vi "TreeItem.Property.Get.vi"(6 "Custom Device Path":string, 8 "error in (no error)":errorcluster, 9 "Default Value":variant, 10 "Property Name":string, 11 "Basenode":refnum<k24>) -> (0 "error out":errorcluster, 1 "Variant":variant, 2 "Found?":bool, 3 "Basenode":refnum<k24>)   [LabVIEW 2017, in "Advanced System Definition.lvlib"]
uses:
  SysDef API/Advanced System Definition.lvlib
  NationalInstruments.VeriStand.SystemStorage
  _Types/Property.DependentFile.ctl
  NationalInstruments.VeriStand
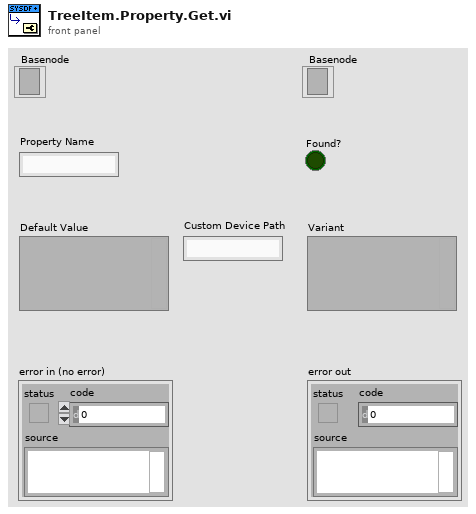
[diagram p1: front panel]
types:
  T1 = typedef "Advanced System Definition.lvlib/Property.DependentFile.ctl" = cluster{"Original Path":path, "Version":string, "RTDestination":path, "ForceDownload":bool, "SupportedTarget":string, "MD5":string}
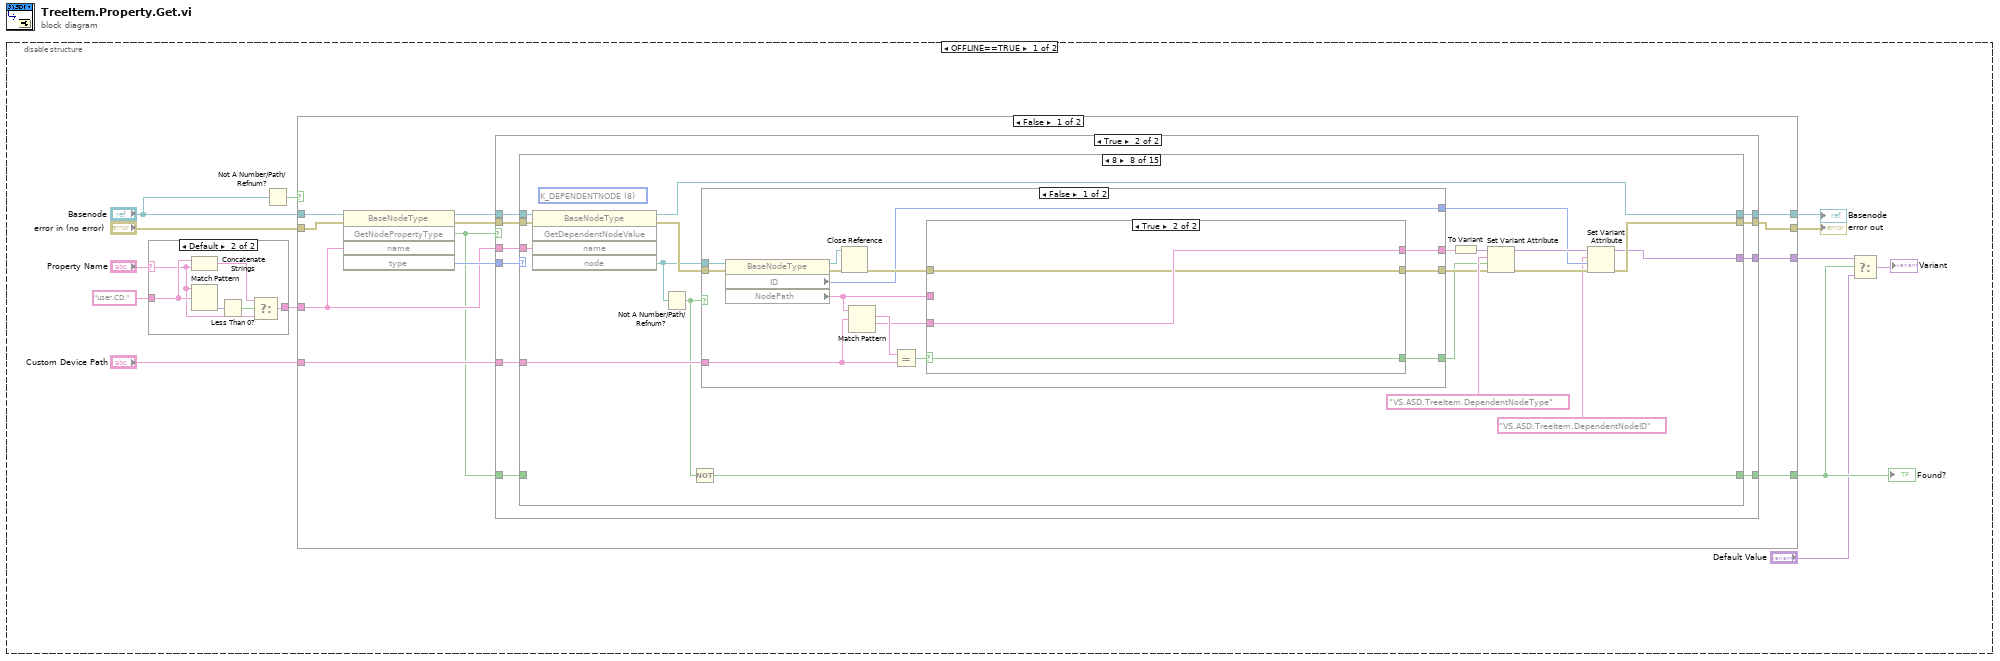
[diagram p0: block diagram]
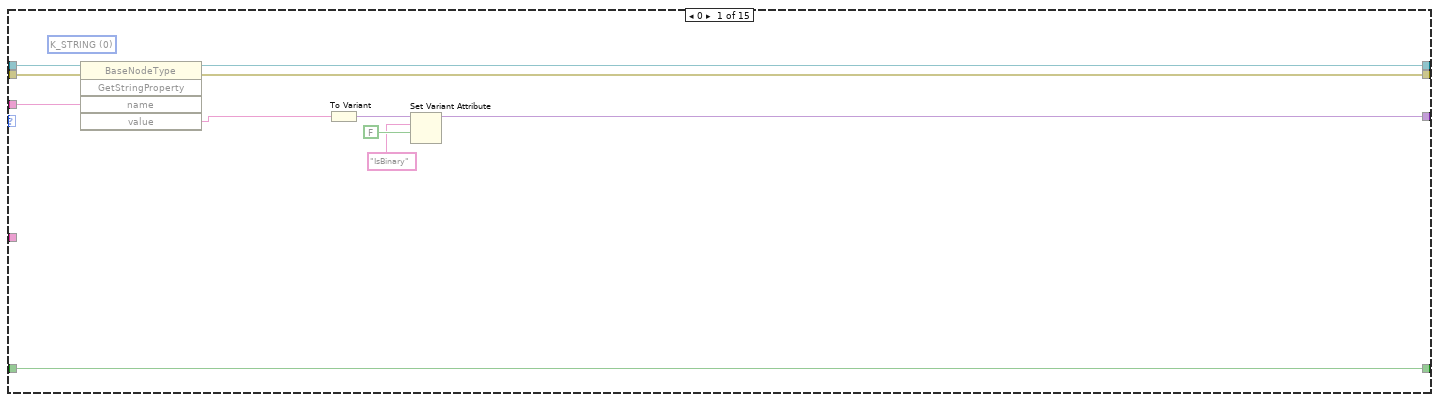
[diagram p4: hidden frame]
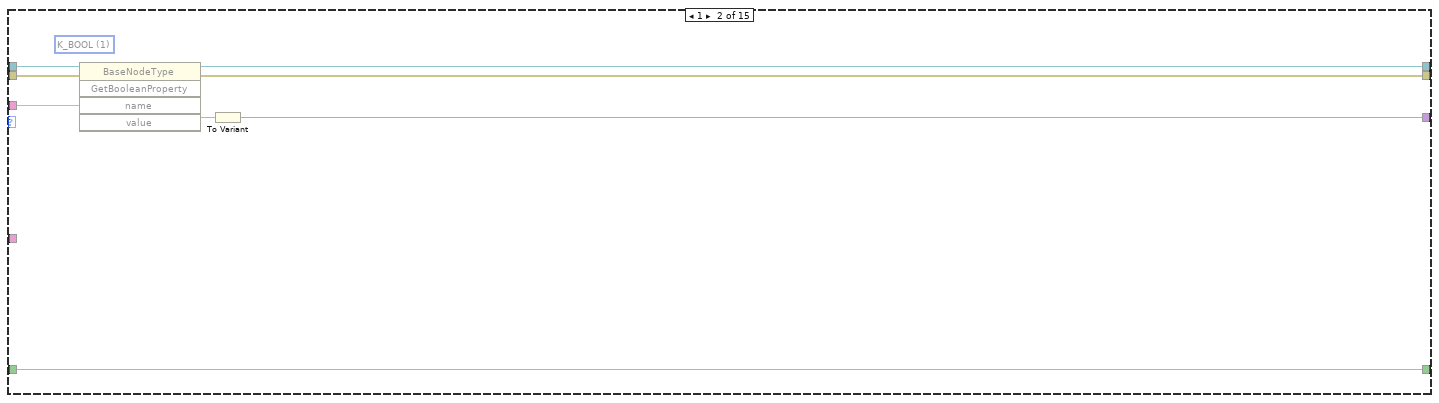
[diagram p5: hidden frame]
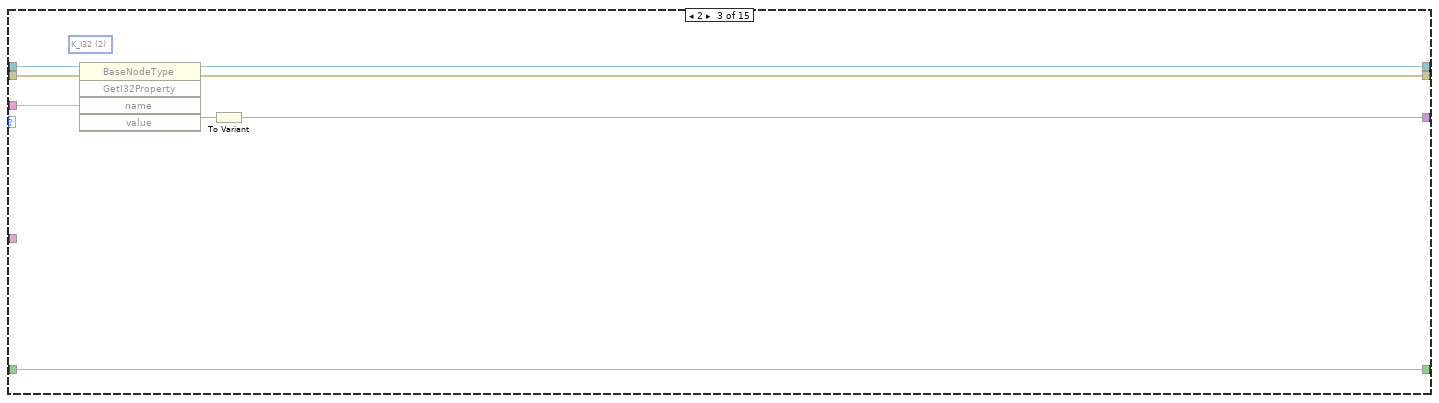
[diagram p6: hidden frame]
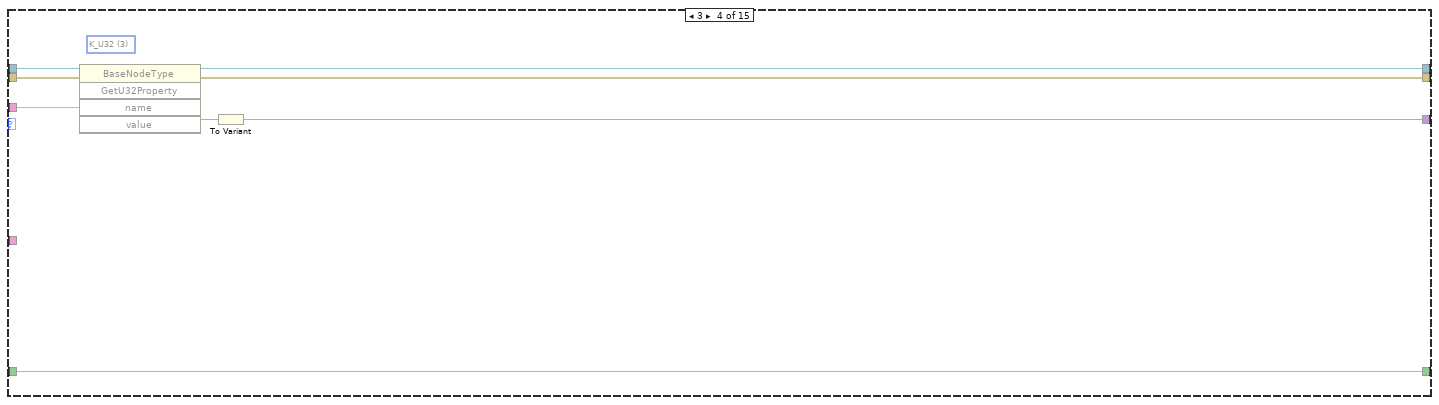
[diagram p7: hidden frame]
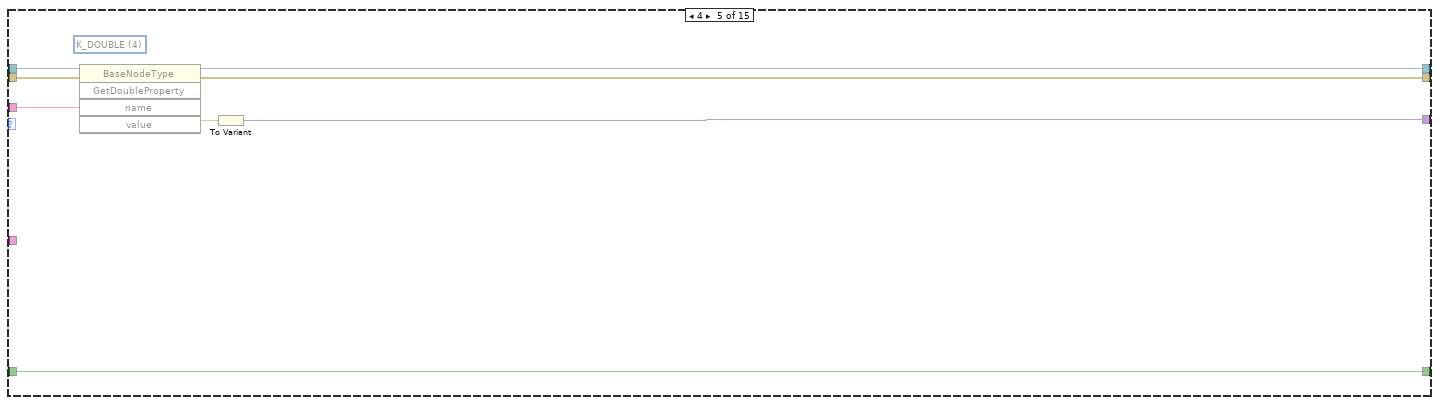
[diagram p8: hidden frame]
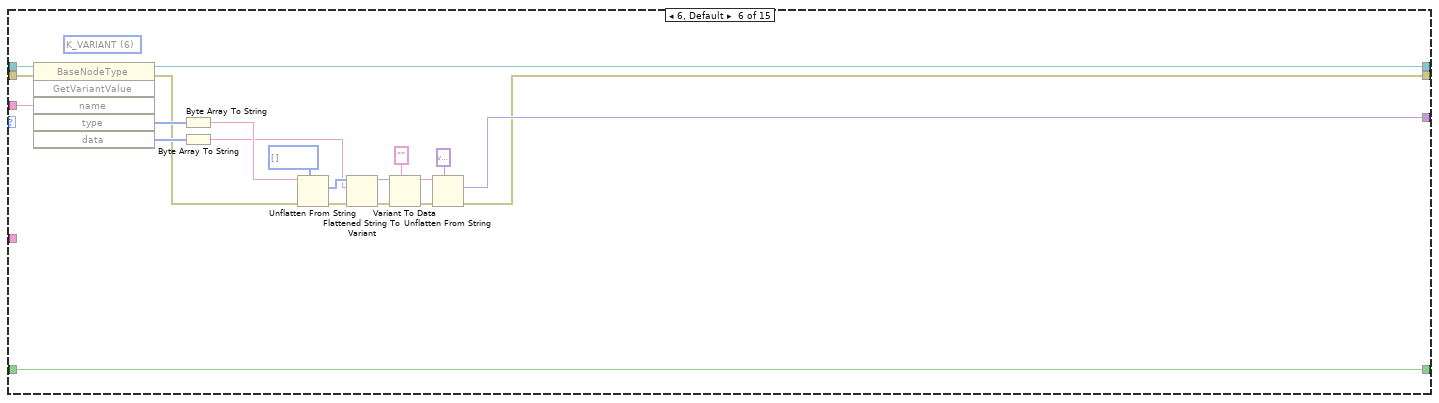
[diagram p9: hidden frame]
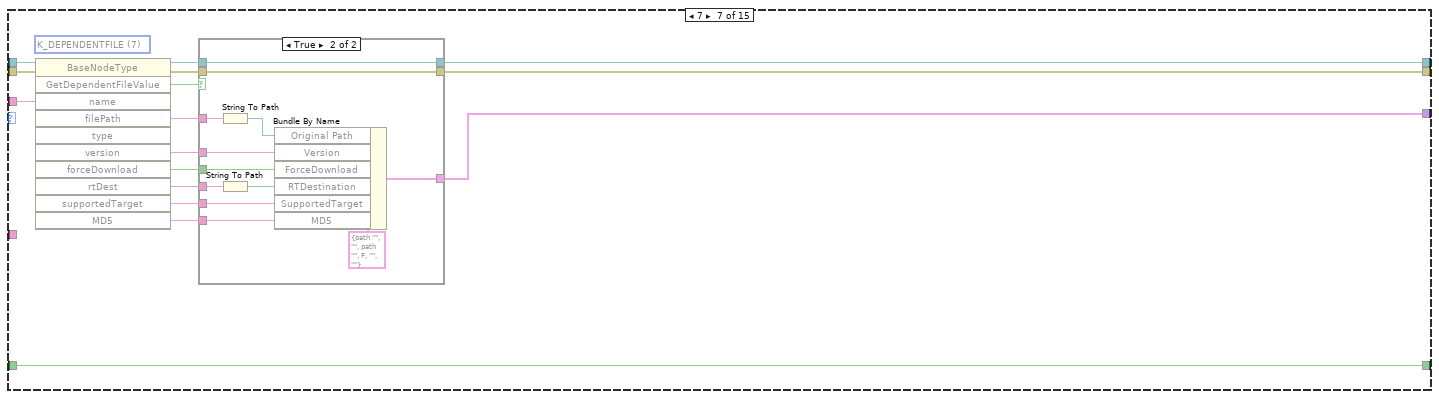
[diagram p10: hidden frame]
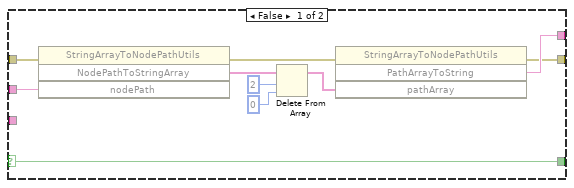
[diagram p12: hidden frame]
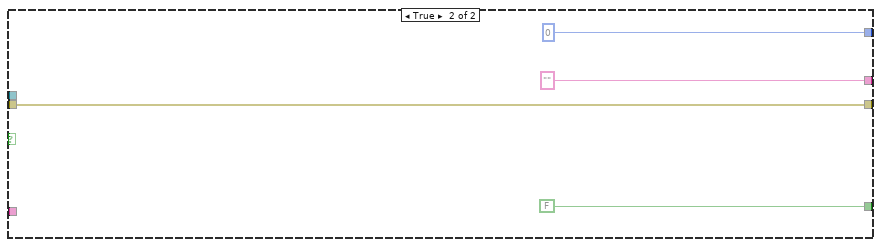
[diagram p13: hidden frame]
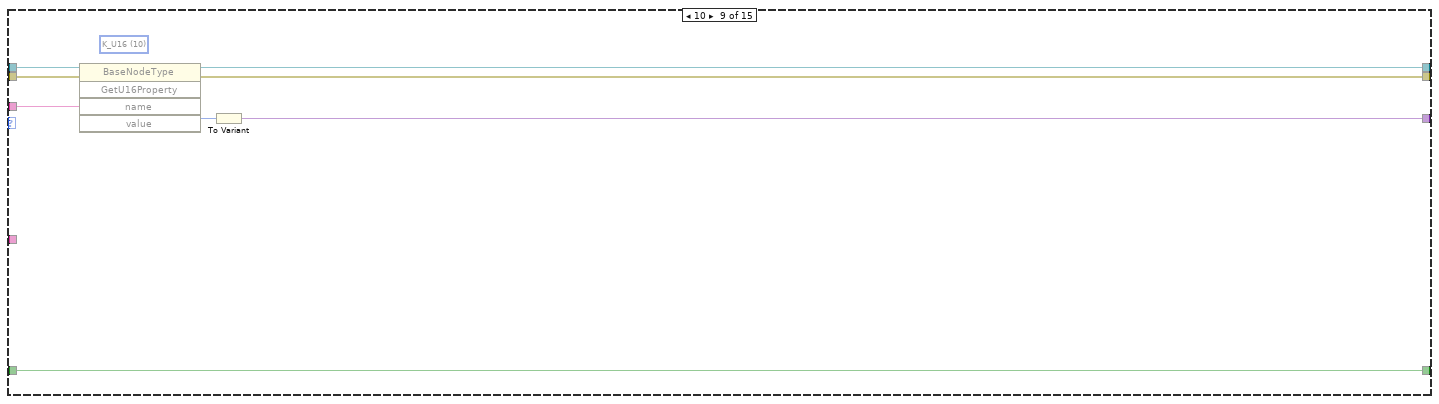
[diagram p14: hidden frame]
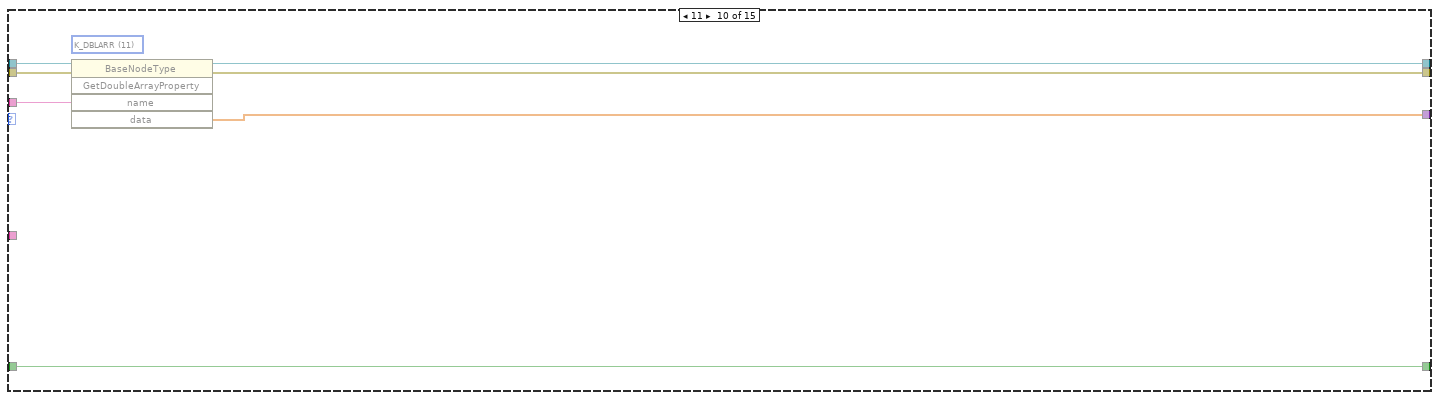
[diagram p15: hidden frame]
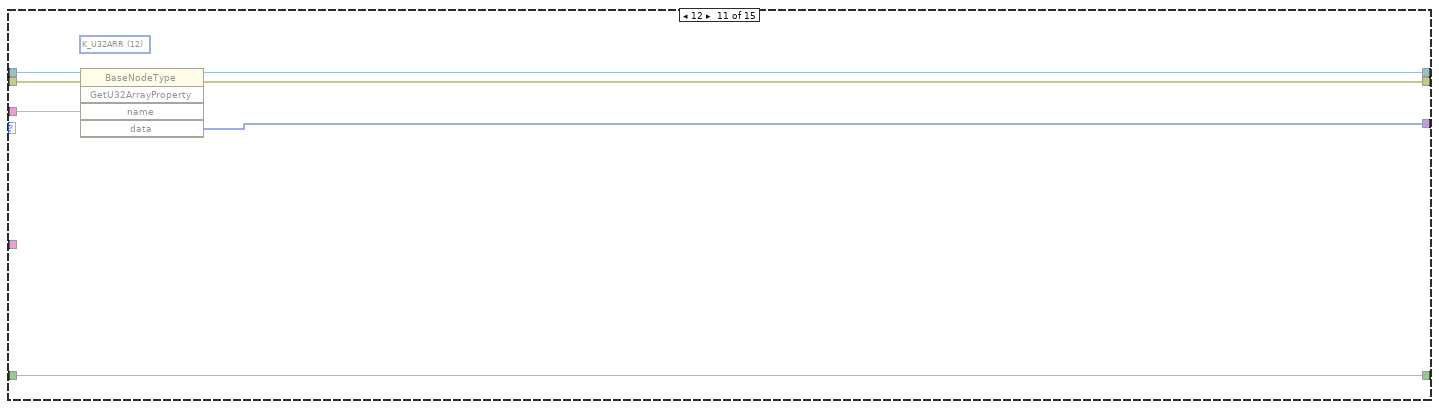
[diagram p16: hidden frame]
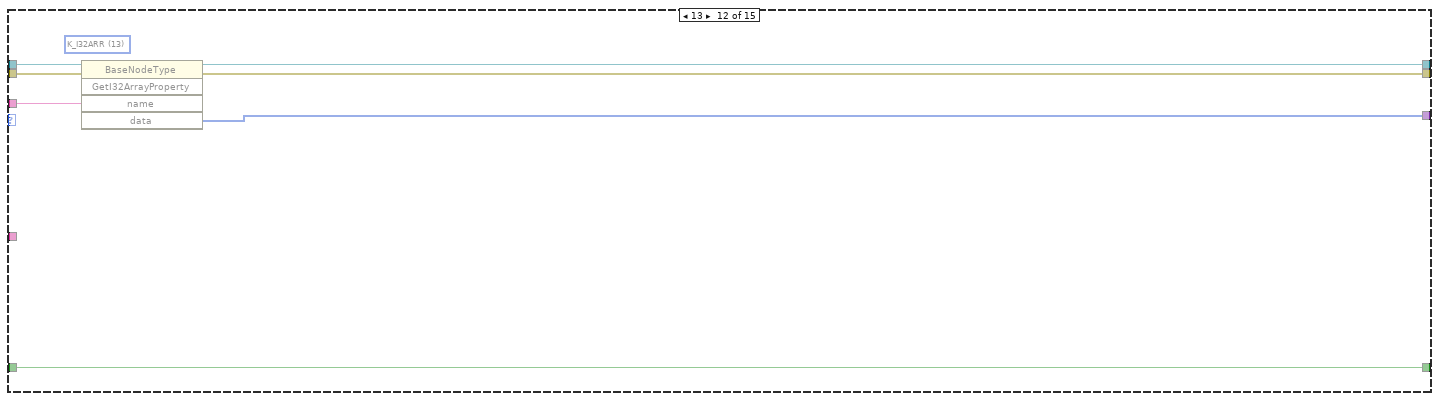
[diagram p17: hidden frame]
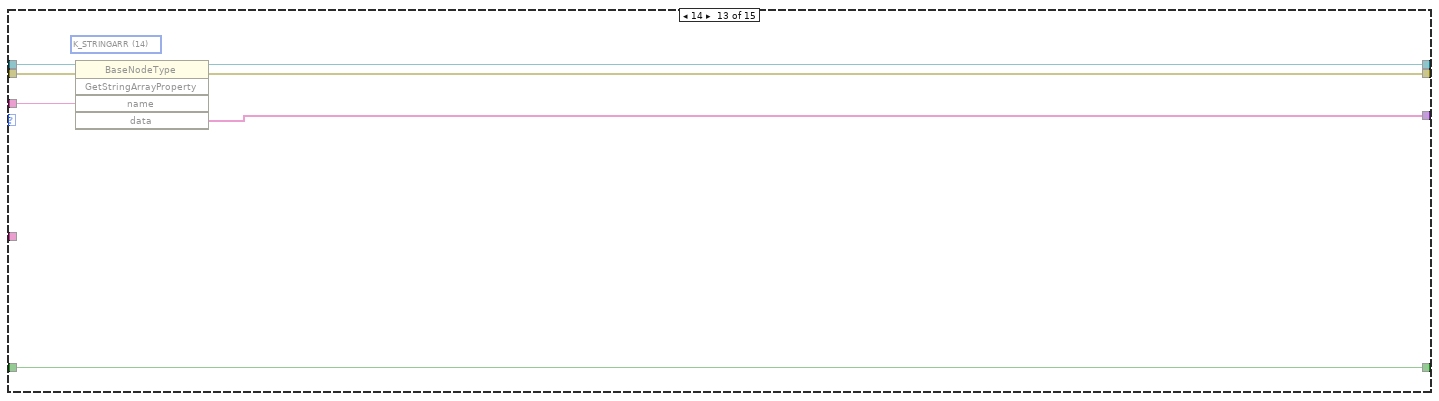
[diagram p18: hidden frame]
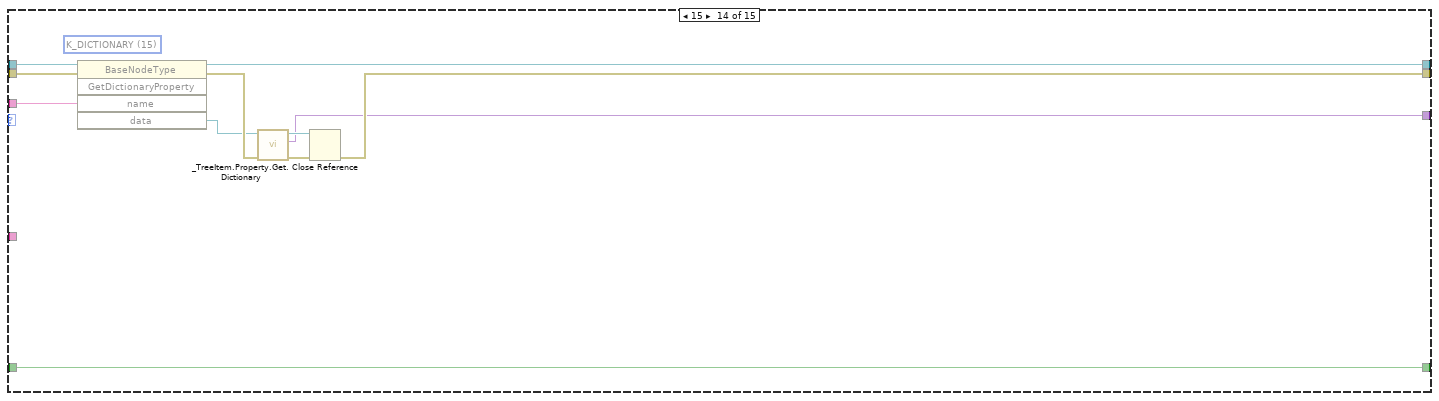
[diagram p19: hidden frame]
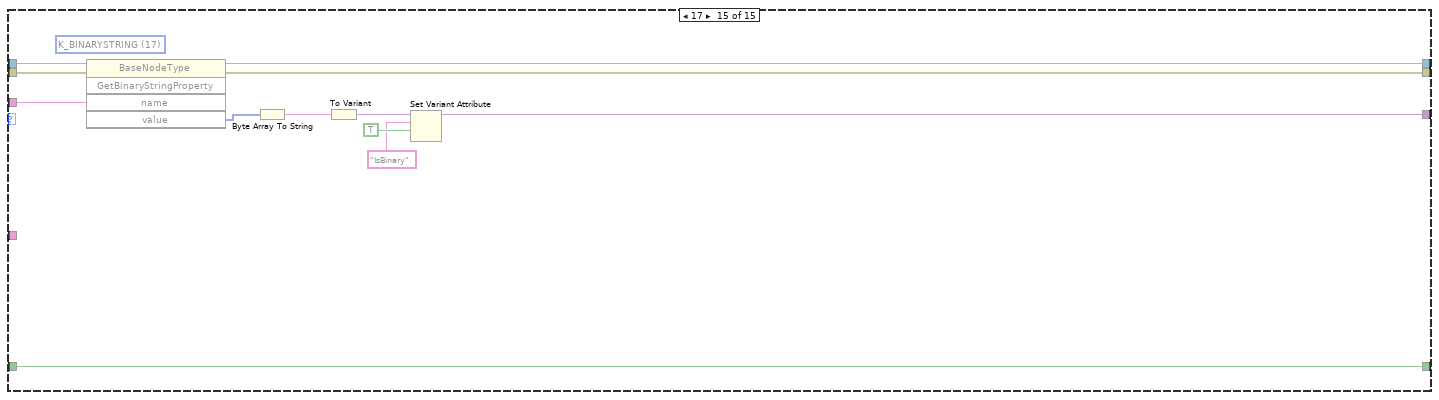
[diagram p20: hidden frame]
diagram:
  n1 = disable-structure shown="OFFLINE==TRUE" {
    frame condition #0 {
      n2 = case shown="Default" "Property Name" {
        selector: "Property Name" -> [w14 w15]
        tunnel: "user.CD." ("regular expression") -> [_ w18]
        tunnel: [w14 w16] -> w3
        frame "Value Table" {
        }
        frame Default {
          n3 = Concatenate Strings(w18, w15) -> (w19:string)
          n4 = Match Pattern(string=w15, regular expression=w18) -> (offset past match=w20:i32)  [unwired: 1 in, 3 out]
          n5 = Less Than 0?(x=w20) -> (x < 0?=w17:bool)
          n6 = Select(t=w19, s=w17, f=w15) -> (s? t:f=w16:string)
        }
      }
      n7 = Not A Number/Path/Refnum?(number/path/refnum="Basenode") -> (NaN/Path/Refnum?=w13:bool)
      n8 = case shown="False" w13 {
        tunnel: w3 -> [w24 _]
        tunnel: "Basenode" -> [w32 w251]
        tunnel: "error in (no error)" -> [w31 w250]
        tunnel: [w21 _] -> w10
        tunnel: [w27 _] -> w9
        tunnel: [w26 w251] -> w6
        tunnel: [w25 w250] -> w5
        tunnel: "Custom Device Path" -> [w23 _]
        frame False {
          n9 = invoke class="BaseNodeType" method="GetNodePropertyType"(reference=w32, error in=w31, "name"=w24) -> (reference out=w28:refnum<k24>, error out=w30:errorcluster, "GetNodePropertyType"=w22:bool, "type"=w29:i32)  [unwired: 2 in, 1 out]
          n10 = case shown="True" w22 {
            tunnel: [w34 w45] -> w26
            tunnel: [w35 w44] -> w25
            tunnel: [_ w43] -> w27
            tunnel: w30 -> [w35 w42]
            tunnel: w29 -> [_ w41]
            tunnel: w28 -> [w34 w40]
            tunnel: w24 -> [_ w39]
            tunnel: w23 -> [_ w38]
            tunnel: [w33 w37] -> w21
            tunnel: w22 -> [w33 w36]
            frame False {
            }
            frame True {
              n11 = case shown="8" w41 {
                tunnel: [w56 w64 w72 w80 w88 w109 w112 w156 w198 w205 w212 w219 w222 w236 w244] -> w45
                tunnel: w42 -> [w55 w63 w71 w79 w87 w108 w121 w159 w197 w204 w211 w218 w226 w237 w248]
                tunnel: [w54 w62 w70 w78 w86 w91 w113 w144 w196 w203 w210 w217 w225 w231 w245] -> w44
                tunnel: [w47 w60 w68 w76 w84 w92 w111 w142 w194 w202 w209 w216 w224 w229 w239] -> w43
                tunnel: w40 -> [w52 w59 w66 w74 w82 w107 w122 w158 w193 w200 w208 w215 w221 w235 w249]
                tunnel: w39 -> [w53 w58 w67 w75 w83 w106 w120 w157 w192 w201 w207 w214 w223 w228 w247]
                tunnel: w38 -> [_ _ _ _ _ _ _ w151 _ _ _ _ _ _ _]
                tunnel: [w46 w57 w65 w73 w81 w89 w110 w146 w191 w199 w206 w213 w220 w227 w238] -> w37
                tunnel: w36 -> [w46 w57 w65 w73 w81 w89 w110 _ w191 w199 w206 w213 w220 w227 w238]
                frame 0 {
                  (unwired) 0 items=["K_STRING", "K_BOOL", "K_I32", "K_U32", "K_DOUBLE", "K_U64", "K_VARIANT", "K_DEPENDENTFILE", "K_DEPENDENTNODE", "K_DATASOURCENODE", "K_U16", "K_DBLARR", "K_U32ARR", "K_I32ARR", "K_STRINGARR", "K_DICTIONARY", "K_DICTIONARYARR"] ("type")
                  n12 = invoke class="BaseNodeType" method="GetStringProperty"(reference=w52, error in=w55, "name"=w53) -> (reference out=w56:refnum<k24>, error out=w54:errorcluster, "value"=w48:string)  [unwired: 2 in, 2 out]
                  n13 = To Variant(anything=w48) -> (Variant=w49:variant)
                  n14 = Set Variant Attribute(Variant=w49, name="IsBinary", value=FALSE ("Set String as Binary")) -> (Variant out=w47:variant)  [unwired: 1 in, 2 out]
                }
                frame 1 {
                  (unwired) 1 items=["K_STRING", "K_BOOL", "K_I32", "K_U32", "K_DOUBLE", "K_U64", "K_VARIANT", "K_DEPENDENTFILE", "K_DEPENDENTNODE", "K_DATASOURCENODE", "K_U16", "K_DBLARR", "K_U32ARR", "K_I32ARR", "K_STRINGARR", "K_DICTIONARY", "K_DICTIONARYARR"] ("type")
                  n15 = invoke class="BaseNodeType" method="GetBooleanProperty"(reference=w59, error in=w63, "name"=w58) -> (reference out=w64:refnum<k24>, error out=w62:errorcluster, "value"=w61:bool)  [unwired: 2 in, 2 out]
                  n16 = To Variant(anything=w61) -> (Variant=w60:variant)
                }
                frame 2 {
                  (unwired) 2 items=["K_STRING", "K_BOOL", "K_I32", "K_U32", "K_DOUBLE", "K_U64", "K_VARIANT", "K_DEPENDENTFILE", "K_DEPENDENTNODE", "K_DATASOURCENODE", "K_U16", "K_DBLARR", "K_U32ARR", "K_I32ARR", "K_STRINGARR", "K_DICTIONARY", "K_DICTIONARYARR"] ("type")
                  n17 = invoke class="BaseNodeType" method="GetI32Property"(reference=w66, error in=w71, "name"=w67) -> (reference out=w72:refnum<k24>, error out=w70:errorcluster, "value"=w69:i32)  [unwired: 2 in, 2 out]
                  n18 = To Variant(anything=w69) -> (Variant=w68:variant)
                }
                frame 3 {
                  (unwired) 3 items=["K_STRING", "K_BOOL", "K_I32", "K_U32", "K_DOUBLE", "K_U64", "K_VARIANT", "K_DEPENDENTFILE", "K_DEPENDENTNODE", "K_DATASOURCENODE", "K_U16", "K_DBLARR", "K_U32ARR", "K_I32ARR", "K_STRINGARR", "K_DICTIONARY", "K_DICTIONARYARR"] ("type")
                  n19 = invoke class="BaseNodeType" method="GetU32Property"(reference=w74, error in=w79, "name"=w75) -> (reference out=w80:refnum<k24>, error out=w78:errorcluster, "value"=w77:u32)  [unwired: 2 in, 2 out]
                  n20 = To Variant(anything=w77) -> (Variant=w76:variant)
                }
                frame 4 {
                  (unwired) 4 items=["K_STRING", "K_BOOL", "K_I32", "K_U32", "K_DOUBLE", "K_U64", "K_VARIANT", "K_DEPENDENTFILE", "K_DEPENDENTNODE", "K_DATASOURCENODE", "K_U16", "K_DBLARR", "K_U32ARR", "K_I32ARR", "K_STRINGARR", "K_DICTIONARY", "K_DICTIONARYARR"] ("type")
                  n21 = invoke class="BaseNodeType" method="GetDoubleProperty"(reference=w82, error in=w87, "name"=w83) -> (reference out=w88:refnum<k24>, error out=w86:errorcluster, "value"=w85:dbl)  [unwired: 2 in, 2 out]
                  n22 = To Variant(anything=w85) -> (Variant=w84:variant)
                }
                frame 6, Default {
                  (unwired) 6 items=["K_STRING", "K_BOOL", "K_I32", "K_U32", "K_DOUBLE", "K_U64", "K_VARIANT", "K_DEPENDENTFILE", "K_DEPENDENTNODE", "K_DATASOURCENODE", "K_U16", "K_DBLARR", "K_U32ARR", "K_I32ARR", "K_STRINGARR", "K_DICTIONARY", "K_DICTIONARYARR"] ("type")
                  n23 = invoke class="BaseNodeType" method="GetVariantValue"(reference=w107, error in=w108, "name"=w106) -> (reference out=w109:refnum<k24>, error out=w90:errorcluster, "type"=w93:u8[], "data"=w94:u8[])  [unwired: 3 in, 2 out]
                  n24 = Byte Array To String(unsigned byte array=w93) -> (string=w102:string)
                  n25 = Byte Array To String(unsigned byte array=w94) -> (string=w101:string)
                  n26 = Unflatten From String(type=i16[] [] ("type string"), binary string=w102, error in (no error)=w90) -> (value=w104:i16[], error out=w103:errorcluster)  [unwired: 2 in, 1 out]
                  n27 = Flattened String To Variant(4:w103, 6:w101, 7:w104) -> (0:w97:errorcluster, 3:w100:variant)
                  n28 = Variant To Data(error in=w97, type="", Variant=w100) -> (data=w98:string, error out=w96:errorcluster)
                  n29 = Unflatten From String(type=variant ("variant"), binary string=w98, error in (no error)=w96) -> (value=w92:variant, error out=w91:errorcluster)  [unwired: 2 in, 1 out]
                }
                frame 7 {
                  (unwired) 7 items=["K_STRING", "K_BOOL", "K_I32", "K_U32", "K_DOUBLE", "K_U64", "K_VARIANT", "K_DEPENDENTFILE", "K_DEPENDENTNODE", "K_DATASOURCENODE", "K_U16", "K_DBLARR", "K_U32ARR", "K_I32ARR", "K_STRINGARR", "K_DICTIONARY", "K_DICTIONARYARR"] ("type")
                  n30 = invoke class="BaseNodeType" method="GetDependentFileValue"(reference=w122, error in=w121, "name"=w120) -> (reference out=w124:refnum<k24>, error out=w123:errorcluster, "GetDependentFileValue"=w125:bool, "filePath"=w119:string, "version"=w118:string, "forceDownload"=w116:bool, "rtDest"=w117:string, "supportedTarget"=w115:string, "MD5"=w114:string)  [unwired: 8 in, 2 out]
                  n31 = case shown="True" w125 {
                    tunnel: [w126 w130] -> w113
                    tunnel: [w127 w136] -> w112
                    tunnel: [_ w139] -> w111
                    tunnel: w123 -> [w126 w130]
                    tunnel: w124 -> [w127 w136]
                    tunnel: w119 -> [_ w135]
                    tunnel: w118 -> [_ w134]
                    tunnel: w117 -> [_ w133]
                    tunnel: w116 -> [_ w129]
                    tunnel: w115 -> [_ w132]
                    tunnel: w114 -> [_ w131]
                    frame False {
                    }
                    frame True {
                      n32 = String To Path(string=w135) -> (path=w128:path)
                      n33 = String To Path(string=w133) -> (path=w137:path)
                      n34 = Bundle By Name(cluster=T1 {"Original Path"=path "", "Version"="", "RTDestination"=path "", "ForceDownload"=FALSE, "SupportedTarget"="", "MD5"=""} ("OptionalInfo"), "Original Path"=w128, "Version"=w134, "ForceDownload"=w129, "RTDestination"=w137, "SupportedTarget"=w132, "MD5"=w131) -> (w139:T1)
                    }
                  }
                }
                frame 8 {
                  (unwired) 8 items=["K_STRING", "K_BOOL", "K_I32", "K_U32", "K_DOUBLE", "K_U64", "K_VARIANT", "K_DEPENDENTFILE", "K_DEPENDENTNODE", "K_DATASOURCENODE", "K_U16", "K_DBLARR", "K_U32ARR", "K_I32ARR", "K_STRINGARR", "K_DICTIONARY", "K_DICTIONARYARR"] ("type")
                  n35 = invoke class="BaseNodeType" method="GetDependentNodeValue"(reference=w158, error in=w159, "name"=w157) -> (reference out=w156:refnum<k24>, error out=w153:errorcluster, "node"=w152:refnum<k24>)  [unwired: 2 in, 2 out]
                  n36 = Not A Number/Path/Refnum?(number/path/refnum=w152) -> (NaN/Path/Refnum?=w147:bool)
                  n37 = Not(x=w147) -> (.not. x?=w146:bool)
                  n38 = case shown="False" w147 {
                    tunnel: w153 -> [w170 w190]
                    tunnel: [w163 w190] -> w149
                    tunnel: w152 -> [w171 _]
                    tunnel: w151 -> [w168 _]
                    tunnel: [w162 "" ("NodePath")] -> w150
                    tunnel: [w161 FALSE] -> w148
                    tunnel: [w160 u64 0 ("ID")] -> w141
                    frame False {
                      n39 = property class="BaseNodeType"(reference=w171, error in=w170) -> (reference out=w172:refnum<k24>, error out=w173:errorcluster, "ID"=w160:u64, "NodePath"=w165:string)
                      n40 = Close Reference(reference=w172, error in (no error)=w173) -> (error out=w164:errorcluster)
                      n41 = Match Pattern(string=w165, regular expression=w168) -> (match substring=w169:string, after substring=w166:string)  [unwired: 1 in, 2 out]
                      n42 = Equal?(x=w169, y=w168) -> (x = y?=w167:bool)
                      n43 = case shown="True" w167 {
                        selector: w167 -> [w183 w185]
                        tunnel: [w183 w185] -> w161
                        tunnel: [w175 w186] -> w162
                        tunnel: w166 -> [_ w186]
                        tunnel: w165 -> [w182 _]
                        tunnel: w164 -> [w176 w184]
                        tunnel: [w174 w184] -> w163
                        frame False {
                          n44 = invoke class="StringArrayToNodePathUtils" method="NodePathToStringArray"(error in=w176, "nodePath"=w182) -> (error out=w177:errorcluster, "NodePathToStringArray"=w181:string[])  [unwired: 2 in, 2 out]
                          n45 = Delete From Array(array=w181, length=2, index=0) -> (array with subset deleted=w178:string[])  [unwired: 1 out]
                          n46 = invoke class="StringArrayToNodePathUtils" method="PathArrayToString"(error in=w177, "pathArray"=w178) -> (error out=w174:errorcluster, "PathArrayToString"=w175:string)  [unwired: 2 in, 2 out]
                        }
                        frame True {
                        }
                      }
                    }
                    frame True {
                    }
                  }
                  n47 = To Variant(anything=w150) -> (Variant=w155:variant)
                  n48 = Set Variant Attribute(Variant=w155, name="VS.ASD.TreeItem.DependentNodeType", value=w148, error in=w149) -> (Variant out=w143:variant, error out=w145:errorcluster)  [unwired: 1 out]
                  n49 = Set Variant Attribute(Variant=w143, name="VS.ASD.TreeItem.DependentNodeID", value=w141, error in=w145) -> (Variant out=w142:variant, error out=w144:errorcluster)  [unwired: 1 out]
                }
                frame 10 {
                  (unwired) 10 items=["K_STRING", "K_BOOL", "K_I32", "K_U32", "K_DOUBLE", "K_U64", "K_VARIANT", "K_DEPENDENTFILE", "K_DEPENDENTNODE", "K_DATASOURCENODE", "K_U16", "K_DBLARR", "K_U32ARR", "K_I32ARR", "K_STRINGARR", "K_DICTIONARY", "K_DICTIONARYARR"] ("type")
                  n50 = invoke class="BaseNodeType" method="GetU16Property"(reference=w193, error in=w197, "name"=w192) -> (reference out=w198:refnum<k24>, error out=w196:errorcluster, "value"=w195:u16)  [unwired: 2 in, 2 out]
                  n51 = To Variant(anything=w195) -> (Variant=w194:variant)
                }
                frame 11 {
                  (unwired) 11 items=["K_STRING", "K_BOOL", "K_I32", "K_U32", "K_DOUBLE", "K_U64", "K_VARIANT", "K_DEPENDENTFILE", "K_DEPENDENTNODE", "K_DATASOURCENODE", "K_U16", "K_DBLARR", "K_U32ARR", "K_I32ARR", "K_STRINGARR", "K_DICTIONARY", "K_DICTIONARYARR"] ("type")
                  n52 = invoke class="BaseNodeType" method="GetDoubleArrayProperty"(reference=w200, error in=w204, "name"=w201) -> (reference out=w205:refnum<k24>, error out=w203:errorcluster, "data"=w202:dbl[])  [unwired: 2 in, 2 out]
                }
                frame 12 {
                  (unwired) 12 items=["K_STRING", "K_BOOL", "K_I32", "K_U32", "K_DOUBLE", "K_U64", "K_VARIANT", "K_DEPENDENTFILE", "K_DEPENDENTNODE", "K_DATASOURCENODE", "K_U16", "K_DBLARR", "K_U32ARR", "K_I32ARR", "K_STRINGARR", "K_DICTIONARY", "K_DICTIONARYARR"] ("type")
                  n53 = invoke class="BaseNodeType" method="GetU32ArrayProperty"(reference=w208, error in=w211, "name"=w207) -> (reference out=w212:refnum<k24>, error out=w210:errorcluster, "data"=w209:u32[])  [unwired: 2 in, 2 out]
                }
                frame 13 {
                  (unwired) 13 items=["K_STRING", "K_BOOL", "K_I32", "K_U32", "K_DOUBLE", "K_U64", "K_VARIANT", "K_DEPENDENTFILE", "K_DEPENDENTNODE", "K_DATASOURCENODE", "K_U16", "K_DBLARR", "K_U32ARR", "K_I32ARR", "K_STRINGARR", "K_DICTIONARY", "K_DICTIONARYARR"] ("type")
                  n54 = invoke class="BaseNodeType" method="GetI32ArrayProperty"(reference=w215, error in=w218, "name"=w214) -> (reference out=w219:refnum<k24>, error out=w217:errorcluster, "data"=w216:i32[])  [unwired: 2 in, 2 out]
                }
                frame 14 {
                  (unwired) 14 items=["K_STRING", "K_BOOL", "K_I32", "K_U32", "K_DOUBLE", "K_U64", "K_VARIANT", "K_DEPENDENTFILE", "K_DEPENDENTNODE", "K_DATASOURCENODE", "K_U16", "K_DBLARR", "K_U32ARR", "K_I32ARR", "K_STRINGARR", "K_DICTIONARY", "K_DICTIONARYARR"] ("type")
                  n55 = invoke class="BaseNodeType" method="GetStringArrayProperty"(reference=w221, error in=w226, "name"=w223) -> (reference out=w222:refnum<k24>, error out=w225:errorcluster, "data"=w224:string[])  [unwired: 2 in, 2 out]
                }
                frame 15 {
                  (unwired) 15 items=["K_STRING", "K_BOOL", "K_I32", "K_U32", "K_DOUBLE", "K_U64", "K_VARIANT", "K_DEPENDENTFILE", "K_DEPENDENTNODE", "K_DATASOURCENODE", "K_U16", "K_DBLARR", "K_U32ARR", "K_I32ARR", "K_STRINGARR", "K_DICTIONARY", "K_DICTIONARYARR"] ("type")
                  n56 = invoke class="BaseNodeType" method="GetDictionaryProperty"(reference=w235, error in=w237, "name"=w228) -> (reference out=w236:refnum<k24>, error out=w234:errorcluster, "data"=w233:refnum<k24>)  [unwired: 2 in, 2 out]
                  n57 = call "_TreeItem.Property.Get.Dictionary.vi"("error in (no error)"=w234, "DictionaryProperty"=w233) -> ("error out"=w232:errorcluster, "Dictionary Variant"=w229:variant, "DictionaryProperty out"=w230:refnum<k24>)  [unwired: 7 in]
                  n58 = Close Reference(reference=w230, error in (no error)=w232) -> (error out=w231:errorcluster)
                }
                frame 17 {
                  (unwired) 17 items=["K_STRING", "K_BOOL", "K_I32", "K_U32", "K_DOUBLE", "K_U64", "K_VARIANT", "K_DEPENDENTFILE", "K_DEPENDENTNODE", "K_DATASOURCENODE", "K_U16", "K_DBLARR", "K_U32ARR", "K_I32ARR", "K_STRINGARR", "K_DICTIONARY", "K_DICTIONARYARR", "K_BINARYSTRING"] ("type")
                  n59 = invoke class="BaseNodeType" method="GetBinaryStringProperty"(reference=w249, error in=w248, "name"=w247) -> (reference out=w244:refnum<k24>, error out=w245:errorcluster, "value"=w246:u8[])  [unwired: 2 in, 2 out]
                  n60 = Byte Array To String(unsigned byte array=w246) -> (string=w240:string)
                  n61 = To Variant(anything=w240) -> (Variant=w241:variant)
                  n62 = Set Variant Attribute(Variant=w241, name="IsBinary", value=TRUE ("Set String as Binary")) -> (Variant out=w239:variant)  [unwired: 1 in, 2 out]
                }
              }
            }
          }
        }
        frame True {
        }
      }
      "Basenode" <- w6
      "Found?" <- w10
      "error out" <- w5
      n63 = Select(t=w9, s=w10, f="Default Value") -> (s? t:f=→"Variant":variant)
    }
    frame condition #1 (active) {
    }
  }
